vi "NanotecSMCPDDriver.get limit switch props.vi"(0 "VISA resource name":refnum<visa-resource-name>, 1 "contollerID":i32=-1, 5 "error in (no error)":errorcluster) -> (14 "VISA resource name out":refnum<visa-resource-name>, 15 "contollerID out":i32=-1, 17 "limitSwitchProperties":bool[](array[boolean]), 19 "error out":errorcluster)   [LabVIEW 2014, in "NanotecSMCPDDriver.lvlib"]
doc: "Gets the properties for the limit switches. This VI should only be used by experts during the commisisioning phase."
uses:
  NanotecSMCPDDriver.lvlib
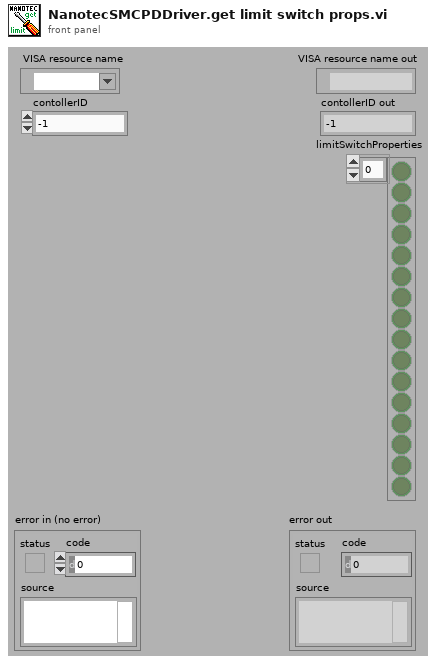
[diagram p1: front panel]
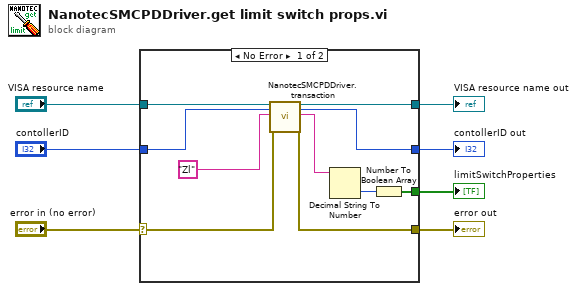
[diagram p0: block diagram]
diagram:
  n1 = case shown="No Error" "error in (no error)" {
    selector: "error in (no error)" -> [w12 w18]
    tunnel: [w14 w20] -> w7
    tunnel: [w13 w18] -> w6
    tunnel: "VISA resource name" -> [w17 w20]
    tunnel: "contollerID" -> [w16 w19]
    tunnel: [w15 w19] -> w3
    tunnel: [w10 _] -> w1
    frame No Error {
      n2 = call "NanotecSMCPDDriver.transaction.vi"("VISAresource"=w17, "contollerID"=w16, "commandString"="Zl", "error in (no error)"=w12) -> ("VISAresource out"=w14:refnum<visa-resource-name>, "contollerID out"=w15:i32, "response"=w11:string, "error out"=w13:errorcluster)  [unwired: 10 in, 2 out]
      n3 = Decimal String To Number(string=w11) -> (number=w8:i32)  [unwired: 2 in, 1 out]
      n4 = Number To Boolean Array(number=w8) -> (Boolean array=w10:bool[])
    }
    frame Error {
    }
  }
  "VISA resource name out" <- w7
  "error out" <- w6
  "contollerID out" <- w3
  "limitSwitchProperties" <- w1
